vi "ManageQMess.vi"(8 "ErrorIn(No Error)":errorcluster caption="entrée d'erreur (pas d'erreur)", 10 "Message":string, 11 "BaseDevice.lvclass":refnum<class "BaseDevice.lvclass">) -> (0 "sortie d'erreur":errorcluster, 3 "BaseDevice.lvclass Out":refnum<class "BaseDevice.lvclass">)   [LabVIEW 2019, in "BaseDevice.lvclass"]
uses:
  BaseDevice.lvclass
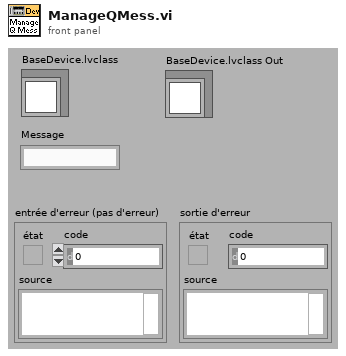
[diagram p1: front panel]
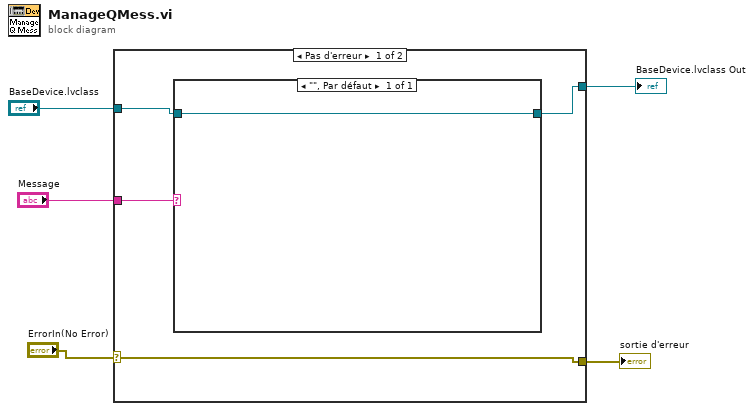
[diagram p0: block diagram]
diagram:
  n1 = case shown="Pas d'erreur" "ErrorIn(No Error)" {
    selector: "ErrorIn(No Error)" -> [w9 w12]
    tunnel: [w9 w12] -> w5
    tunnel: "BaseDevice.lvclass" -> [w7 w11]
    tunnel: [w8 w11] -> w2
    tunnel: "Message" -> [w6 _]
    frame No Error {
      n2 = case shown="\"\", Par défaut" w6 {
        tunnel: [w10] -> w8
        tunnel: w7 -> [w10]
        frame "", Default {
        }
      }
    }
    frame Error {
    }
  }
  "sortie d'erreur" <- w5
  "BaseDevice.lvclass Out" <- w2
